vi "ProdaNG.Tree.Resuls.TestSteps.Add.vi"(6 "Products":T1[](array[typedef]), 7 "TestStepsTree":refnum<vi>, 8 "error in (no error)":errorcluster, 9 "units":T3[](array[typedef]), 10 "Identification":T2, 11 "dbHandleIn":i32) -> (0 "error out":errorcluster, 3 "dbHandle":i32)   [LabVIEW 2016]
doc: "This function returns a product structure for a product, which is identified by a part and a serial number.\nImportant information: The field 'individual' was taken over from the field 'allgemein' of the legacy data directly. Because of this most products have the value 0 further on and only a few the value 1. \nParameter:\nhandle is an Integer, which is returned by the function Login() at the creation of a new connection.\nwabcoPartId is the Id of the part.\nserialNumber is the serial number of the product for the part above.\nproduct is a pointer on a product structure, which is filled if the returncode is 0. The structure must be defined in the calling program.\n\nReturncodes:\n0 No error\n< 0 ORACLE Error code\n6 (ERROR_INVALID_HANDLE) in case of an invalid handle\n1403 Record does not exist"
uses:
  Controls/ProdaNG.UnitSimple.ctl
  Controls/ProdaNG.Product.ctl
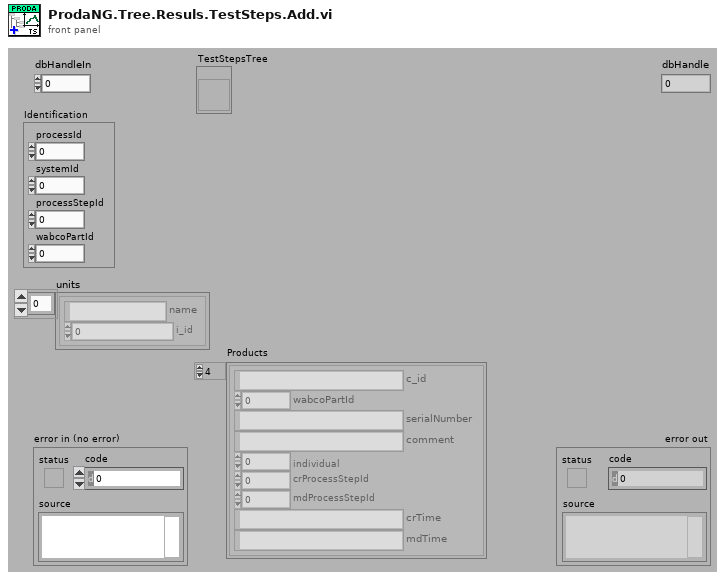
[diagram p1: front panel]
types:
  T1 = typedef "ProdaNG.Product.ctl" = cluster{"c_id":string, "wabcoPartId":i32, "serialNumber":string, "comment":string, "individual":i32, "crProcessStepId":i32, "mdProcessStepId":i32, "crTime":string, "mdTime":string}
  T2 = cluster{"processId":i32, "systemId":i32, "processStepId":i32, "wabcoPartId":i32}
  T3 = typedef "ProdaNG.UnitSimple.ctl" = cluster{"name":string, "i_id":i32}
  T4 = typedef "ProdaNG.TestStep.ctl" = cluster{"i_id":i32, "processStepId":i32, "testSequence":i32, "testOrder":i32, "mdReason":string, "mdUser":string, "mdTime":string, "description":string}
  T5 = typedef "ProdaNG.ProcessResult.ctl" = cluster{"c_id":string, "productId":string, "processId":i32, "statusId":i32, "startTime":string, "endTime":string}
  T6 = typedef "ProdaNG.ProcessStepResult.ctl" = cluster{"c_id":string, "processResultId":string, "processStepId":i32, "statusId":i32, "operatorId":i32, "startTime":string, "endTime":string}
  T7 = typedef "ProdaNG.TestStepResult.ctl" = cluster{"c_id":string, "processStepResultId":string, "testStepId":i32, "statusId":i32}
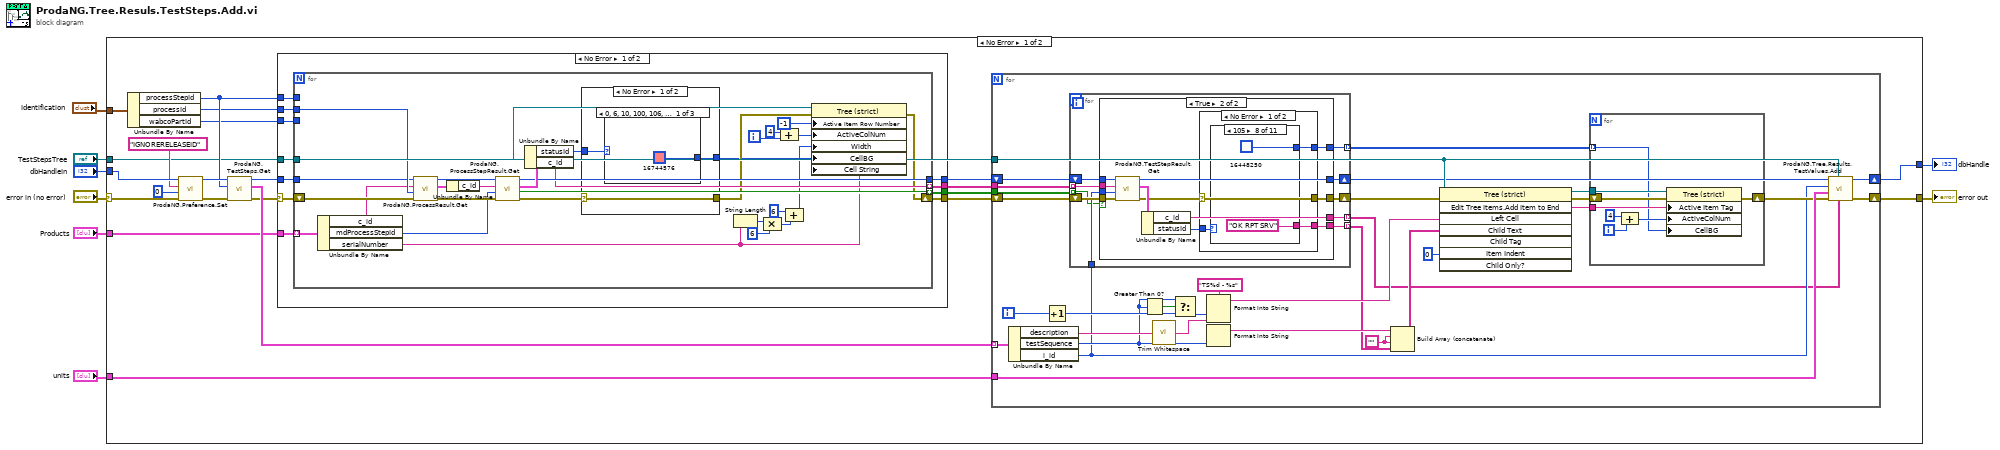
[diagram p0: block diagram]
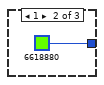
[diagram p2: hidden frame]
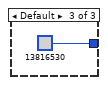
[diagram p3: hidden frame]
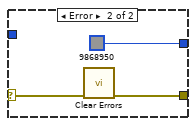
[diagram p4: hidden frame]
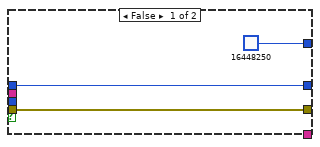
[diagram p6: hidden frame]
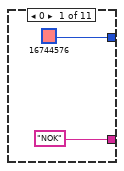
[diagram p7: hidden frame]
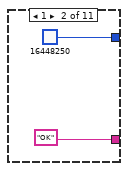
[diagram p8: hidden frame]
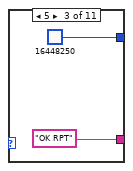
[diagram p9: hidden frame]
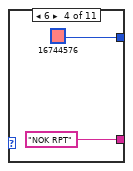
[diagram p10: hidden frame]
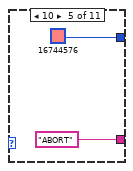
[diagram p11: hidden frame]
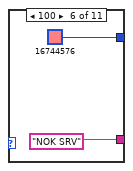
[diagram p12: hidden frame]
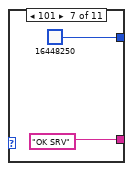
[diagram p13: hidden frame]
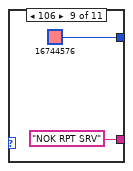
[diagram p14: hidden frame]
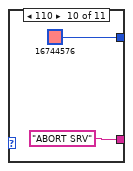
[diagram p15: hidden frame]
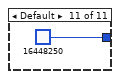
[diagram p16: hidden frame]
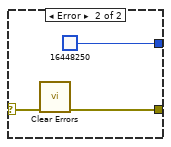
[diagram p17: hidden frame]
diagram:
  n1 = case shown="No Error" "error in (no error)" {
    selector: "error in (no error)" -> [w23 w177]
    tunnel: [w27 w177] -> w5
    tunnel: "dbHandleIn" -> [w26 w176]
    tunnel: [w29 w176] -> w6
    tunnel: "Identification" -> [w22 _]
    tunnel: "TestStepsTree" -> [w10 _]
    tunnel: "units" -> [w30 _]
    tunnel: "Products" -> [w9 _]
    frame No Error {
      n2 = Unbundle By Name(w22) -> ("processStepId"=w17:i32, "processId"=w16:i32, "wabcoPartId"=w15:i32)
      n3 = call "ProdaNG.Preference.Set.vi"("error in"=w23, "value"=0, "key"="IGNORERELEASEID", "dbHandleIn"=w26) -> ("error out"=w20:errorcluster, "dbHandle"=w21:i32)  [unwired: 6 in]
      n4 = call "ProdaNG.TestSteps.Get.vi"("error in (no error)"=w20, "processStepId"=w17, "dbHandleIn"=w21) -> ("error out"=w13:errorcluster, "TestSteps"=w28:T4[], "dbHandle"=w19:i32)  [unwired: 6 in]
      n5 = case shown="No Error" w13 {
        selector: w13 -> [w33 w82]
        tunnel: w19 -> [w41 w81]
        tunnel: [w40 w82] -> w11
        tunnel: [w39 w81] -> w18
        tunnel: w17 -> [w38 _]
        tunnel: w16 -> [w37 _]
        tunnel: w15 -> [w36 _]
        tunnel: [w35 _] -> w14
        tunnel: w9 -> [w34 _]
        tunnel: [w32 _] -> w12
        tunnel: w10 -> [w31 _]
        frame No Error {
          n6 = for {
            tunnel: w41 -> [w52]
            tunnel: [w66] -> w39
            tunnel: w38 -> [_]
            tunnel: w37 -> [w65]
            tunnel: w36 -> [_]
            tunnel: [w62] -> w35 mode=indexing
            shift-right: [w57] -> w40
            shift-left: w33 -> [w50]
            tunnel: w34 -> [w51] mode=indexing
            tunnel: [w64] -> w32 mode=indexing
            tunnel: w31 -> [w53]
            i -> [w58]
            n7 = Unbundle By Name(w51) -> ("c_id"=w48:string, "mdProcessStepId"=w49:i32, "serialNumber"=w47:string)
            n8 = call "ProdaNG.ProcessResult.Get.vi"("error in (no error)"=w50, "processId"=w65, "productId"=w48, "dbHandle"=w52) -> ("error out"=w69:errorcluster, "ProcessResult"=w68:T5, "dbHandle out"=w70:i32)  [unwired: 4 in, 1 out]
            n9 = Unbundle By Name(w68) -> ("c_id"=w71:string)
            n10 = call "ProdaNG.ProcessStepResult.Get.vi"("error in (no error)"=w69, "processStepId"=w49, "processResultId"=w71, "dbHandle"=w70) -> ("error out"=w55:errorcluster, "Found"=w64:bool, "ProcessStepResult"=w67:T6, "dbHandle out"=w66:i32)  [unwired: 4 in]
            n11 = Unbundle By Name(w67) -> ("statusId"=w63:i32, "c_id"=w62:string)
            n12 = case shown="No Error" w55 {
              selector: w55 -> [w72 w80]
              tunnel: w63 -> [w74 _]
              tunnel: [w72 w79] -> w56
              tunnel: [w73 u32 9868950] -> w54
              frame No Error {
                n13 = case shown="0, 6, 10, 100, 106, 110" w74 {
                  tunnel: [u32 16744576 u32 6618880 u32 13816530] -> w73
                  frame 0, 6, 10, 100, 106, 110 {
                  }
                  frame 1 {
                  }
                  frame Default {
                  }
                }
              }
              frame Error {
                n14 = call <vilib>:"Clear Errors.vi"("error in (no error)"=w80) -> ("error out"=w79:errorcluster)  [unwired: 5 in, 1 out]
              }
            }
            n15 = String Length(string=w47) -> (length=w46:i32)
            n16 = Compound Arithmetic op=MULTIPLY(w46, 6 ("value")) -> (w44:i32)
            n17 = Compound Arithmetic op=ADD(4 ("value"), w58) -> (w60:i32)
            n18 = Compound Arithmetic op=ADD(6 ("value"), w44) -> (w42:i32)
            n19 = property class="Tree (strict)"(reference=w53, error in=w56, "Active Item Row Number"=-1 ("Active Item:Row Number"), "ActiveColNum"=w60, "Width"=w42, "CellBG"=w54, "Cell String"=w47) -> (error out=w57:errorcluster)  [unwired: 1 out]
          }
        }
        frame Error {
        }
      }
      n20 = for {
        shift-right: [w112] -> w27
        shift-left: w11 -> [w93]
        tunnel: w28 -> [w97] mode=indexing
        tunnel: w10 -> [w111]
        shift-right: [w107] -> w29
        shift-left: w18 -> [w92]
        tunnel: w30 -> [w110]
        tunnel: w14 -> [w89]
        tunnel: w12 -> [w86]
        i -> [w106]
        w109 = ""
        n21 = Unbundle By Name(w97) -> ("description"=w105:string, "testSequence"=w102:i32, "i_id"=w87:i32)
        n22 = Increment(x=w106) -> (x+1=w103:i32)
        n23 = for {
          shift-right: [w121] -> w90
          shift-left: w93 -> [w124]
          shift-right: [w122] -> w91
          shift-left: w92 -> [w123]
          tunnel: w89 -> [w120] mode=indexing
          tunnel: w87 -> [w119]
          tunnel: w86 -> [w118] mode=indexing
          tunnel: [w117] -> w83 mode=indexing
          tunnel: [w116] -> w85 mode=indexing
          tunnel: [w115] -> w84 mode=indexing
          n24 = case shown="True" w118 {
            tunnel: w124 -> [w126 w139]
            tunnel: w123 -> [w127 w138]
            tunnel: [w127 w137] -> w122
            tunnel: [w126 w131] -> w121
            tunnel: w120 -> [_ w136]
            tunnel: w119 -> [_ w135]
            tunnel: [_ w128] -> w117
            tunnel: [_ w133] -> w116
            tunnel: [u32 16448250 w129] -> w115
            frame False {
            }
            frame True {
              n25 = call "ProdaNG.TestStepResult.Get.vi"("error in (no error)"=w139, "testStepId"=w135, "processStepResulttId"=w136, "dbHandle"=w138) -> ("error out"=w130:errorcluster, "TestStepResult"=w134:T7, "dbHandle out"=w137:i32)  [unwired: 4 in, 1 out]
              n26 = Unbundle By Name(w134) -> ("c_id"=w133:string, "statusId"=w132:i32)
              n27 = case shown="No Error" w130 {
                selector: w130 -> [w140 w167]
                tunnel: w132 -> [w143 _]
                tunnel: [w140 w166] -> w131
                tunnel: [w141 u32 16448250] -> w129
                tunnel: [w142 _] -> w128
                frame No Error {
                  n28 = case shown="105" w143 {
                    tunnel: ["NOK" "OK" "OK RPT" "NOK RPT" "ABORT" "NOK SRV" "OK SRV" "OK RPT SRV" "NOK RPT SRV" "ABORT SRV" _] -> w142
                    tunnel: [u32 16744576 u32 16448250 u32 16448250 u32 16744576 u32 16744576 u32 16744576 u32 16448250 u32 16448250 u32 16744576 u32 16744576 u32 16448250] -> w141
                    frame 0 {
                    }
                    frame 1 {
                    }
                    frame 5 {
                    }
                    frame 6 {
                    }
                    frame 10 {
                    }
                    frame 100 {
                    }
                    frame 101 {
                    }
                    frame 105 {
                    }
                    frame 106 {
                    }
                    frame 110 {
                    }
                    frame Default {
                    }
                  }
                }
                frame Error {
                  n29 = call <vilib>:"Clear Errors.vi"("error in (no error)"=w167) -> ("error out"=w166:errorcluster)  [unwired: 5 in, 1 out]
                }
              }
            }
          }
        }
        n30 = Greater Than 0?(x=w102) -> (x > 0?=w104:bool)
        n31 = call <vilib>:"Trim Whitespace.vi"("string"=w105) -> ("trimmed string"=w88:string)  [unwired: 1 in]
        n32 = Select(t=w102, s=w104, f=w103) -> (s? t:f=w101:i32)
        n33 = Format Into String(format string="TS%d - %s", w101, w88) -> (resulting string=w108:string)  [unwired: 2 in, 1 out]
        n34 = Format Into String(w102) -> (resulting string=w114:string)  [unwired: 3 in, 1 out]
        n35 = Build Array (concatenate)(w114, w109, w109, w83) -> (w113:string[])
        n36 = invoke on="Invoke Node" class="Tree (strict)" method="Edit Tree Items.Add Item to End"(reference=w111, error in=w90, "Left Cell"=w108, "Child Text"=w113, "Item Indent"=0 ("New Item Indentation")) -> (reference out=w98:refnum<vi>, error out=w95:errorcluster, "Edit Tree Items:Add Item to End"=w94:string)  [unwired: 3 in, 5 out]
        n37 = for {
          tunnel: w98 -> [w175]
          tunnel: w94 -> [w172]
          shift-right: [w174] -> w96
          shift-left: w95 -> [w173]
          tunnel: w84 -> [w170] mode=indexing
          i -> [w168]
          n38 = Compound Arithmetic op=ADD(4 ("value"), w168) -> (w171:i32)
          n39 = property class="Tree (strict)"(reference=w175, error in=w173, "Active Item Tag"=w172, "ActiveColNum"=w171, "CellBG"=w170) -> (error out=w174:errorcluster)  [unwired: 1 out]
        }
        n40 = call "ProdaNG.Tree.Results.TestValues.Add.vi"("TestStepResultIDs"=w85, "TestStepsTree"=w111, "error in (no error)"=w96, "units"=w110, "testStepId"=w87, "dbHandleIn"=w91) -> ("error out"=w112:errorcluster, "dbHandle"=w107:i32)  [unwired: 4 in]
      }
    }
    frame Error {
    }
  }
  "error out" <- w5
  "dbHandle" <- w6
